vi "Auto Select Begin.vi"() -> ()   [LabVIEW 2014]
uses:
  <vilib>/Rock Robotics/SystemInterfaces/AI/FPGA_AIChannel.ctl
  <vilib>/Rock Robotics/SystemInterfaces/Typedef/FPGA_TypedefAnalogModule.ctl
panel:
  in  "Analog Channel":T1=enum."AI 1"
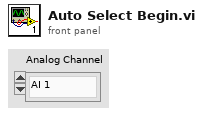
[diagram p1: front panel]
types:
  T1 = typedef "FPGA_AIChannel.ctl" = enum8{"AI 0", "AI 1", "AI 2", "AI 3", "AI MXP 0", "AI MXP 1", "AI MXP 2", "AI MXP 3", "Invalid"}
  T2 = typedef "FPGA_TypedefAnalogModule.ctl" = enum16{"Controller 1"}
  T3 = typedef "WPI_PotentiometerDevRef.ctl" = cluster{"DevStatus":errorcluster, "Controller":T2, "Analog Channel":T1, "Invert Output":bool}
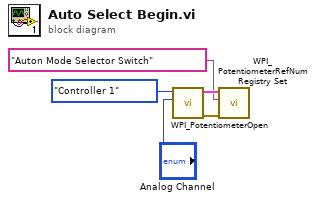
[diagram p0: block diagram]
diagram:
  n1 = call <vilib>:"WPI_PotentiometerOpen.vi"("Analog Channel"="Analog Channel", "Controller"=FPGA_TypedefAnalogModule."Controller 1") -> ("error out"=w5:errorcluster, "PotDevRef"=w4:T3)  [unwired: 8 in]
  n2 = call <vilib>:"WPI_PotentiometerRefNum Registry Set.vi"("error in (no error)"=w5, "refnum name"="Auton Mode Selector Switch", "PotDevRef"=w4) -> ()  [unwired: 7 in, 2 out]
